vi "氨氮测量数据储存.vi"   [LabVIEW 2016, in "斯坦道氨氮.lvlib"]
types:
  T1 = cluster{"时间标识":timestamp, "监测值":sgl, "单位":u16, "数据标识":string, "因子编码":u32, "标样参考值":sgl, "F0":sgl, "F1":sgl, "F2":sgl, "F3":sgl, "F4":sgl, "F5":sgl, "F6":sgl, "F7":sgl, "X":sgl, "温度":sgl, "湿度":sgl, "量程标识":string}
  T2 = enum16{"维护数据", "水样测试", "标样核查", "零点核查", "跨度核查", "空白测试", "平行样测试", "加标回收", "空白校准", "标样校准", "初始化（清洗）"}
  T3 = cluster{"运行模式":enum16{"维护模式", "常规模式", "应急模式", "质控模式"}, "质控频次":enum16{"关闭", "每天", "星期一", "星期二", "星期三", "星期四", "星期五", "星期六", "星期日"}, "空白核查时间":u16, "跨度核查时间":u16, "24H周期设置":bool[]}
  T4 = cluster{"系统时间":timestamp, "工作状态":enum16{"空闲", "水样测试", "标样核查", "零点核查", "跨度核查", "空白测试", "平行样测试", "加标回收", "空白校准", "标样校准", "初始化（清洗）"}, "测量模式":enum16{"待机", "连续模式", "周期模式", "定点模式", "受控模式", "手动模式"}, "告警代码":enum16{"无告警", "缺试剂告警", "缺水样告警", "缺蒸馏水告警", "缺标液告警", "仪表漏液告警", "标定异常告警", "超量程告警", "加热异常", "低试剂预警", "超上限告警", "超下限告警", "仪表内部其他异常", "滴定异常告警", "电极异常告警", "量程切换告警", "参数设置告警", "PH电极电位异常", "电导率电极异常", "浊度光度异常", "溶解氧电极异常", "溶解氧光强异常", "温度异常告警", "PH异常告警", "溶解氧异常告警", "电导率异常告警", "浊度异常告警", "叶绿素异常告警", "藻密度异常告警", "蓝绿藻异常告警", "ORP异常告警", "氨氮异常告警", "清洁刷异常告警", "SD卡异常告警", "蓝牙异常告警", "Wifi异常告警", "流程异常告警"}, "故障代码":enum16{"无故障", "电机故障", "温度故障", "通讯故障", "滴定故障"}, "日志代码":u16, "软件版本":u16, "F0":sgl, "F1":sgl, "F2":sgl, "F3":sgl, "T":sgl, "H":sgl, "id":u16, "flowid":u16, "量程":u16, "总磷控温温度1":sgl, "营养盐控温温度2":sgl, "ADC":sgl}
  T5 = enum16{"空闲", "水样测试", "标样核查", "零点核查", "跨度核查", "空白测试", "平行样测试", "加标回收", "空白校准", "标样校准", "初始化（清洗）"}
  T6 = cluster{"因子编码":u32, "单位":u16, "标样参考值":sgl, "水样数据时间":timestamp, "水样实测值":sgl, "水样数据标识":string, "标样数据时间":timestamp, "标样实测值":sgl, "标样数据标识":string, "空白数据时间":timestamp, "空白实测值":sgl, "空白数据标识":string, "零点核查数据时间":timestamp, "零点核查实测值":sgl, "零点核查数据标识":string, "跨度核查数据时间":timestamp, "跨度核查实测值":sgl, "跨度核查数据标识":string, "加标回收数据时间":timestamp, "加标回收实测值":sgl, "加标回收数据标识":string, "平行样数据时间":timestamp, "平行样实测值":sgl, "平行样数据标识":string, "F0":sgl, "F1":sgl, "F2":sgl, "F3":sgl, "F4":sgl, "F5":sgl, "F6":sgl, "F7":sgl, "温度":sgl, "湿度":sgl, "X值":sgl}
  T7 = cluster{"氨氮跨度值":dbl, "氨氮零点标准液浓度":dbl, "氨氮跨度标准液浓度":dbl, "氨氮标准液标准浓度":dbl}
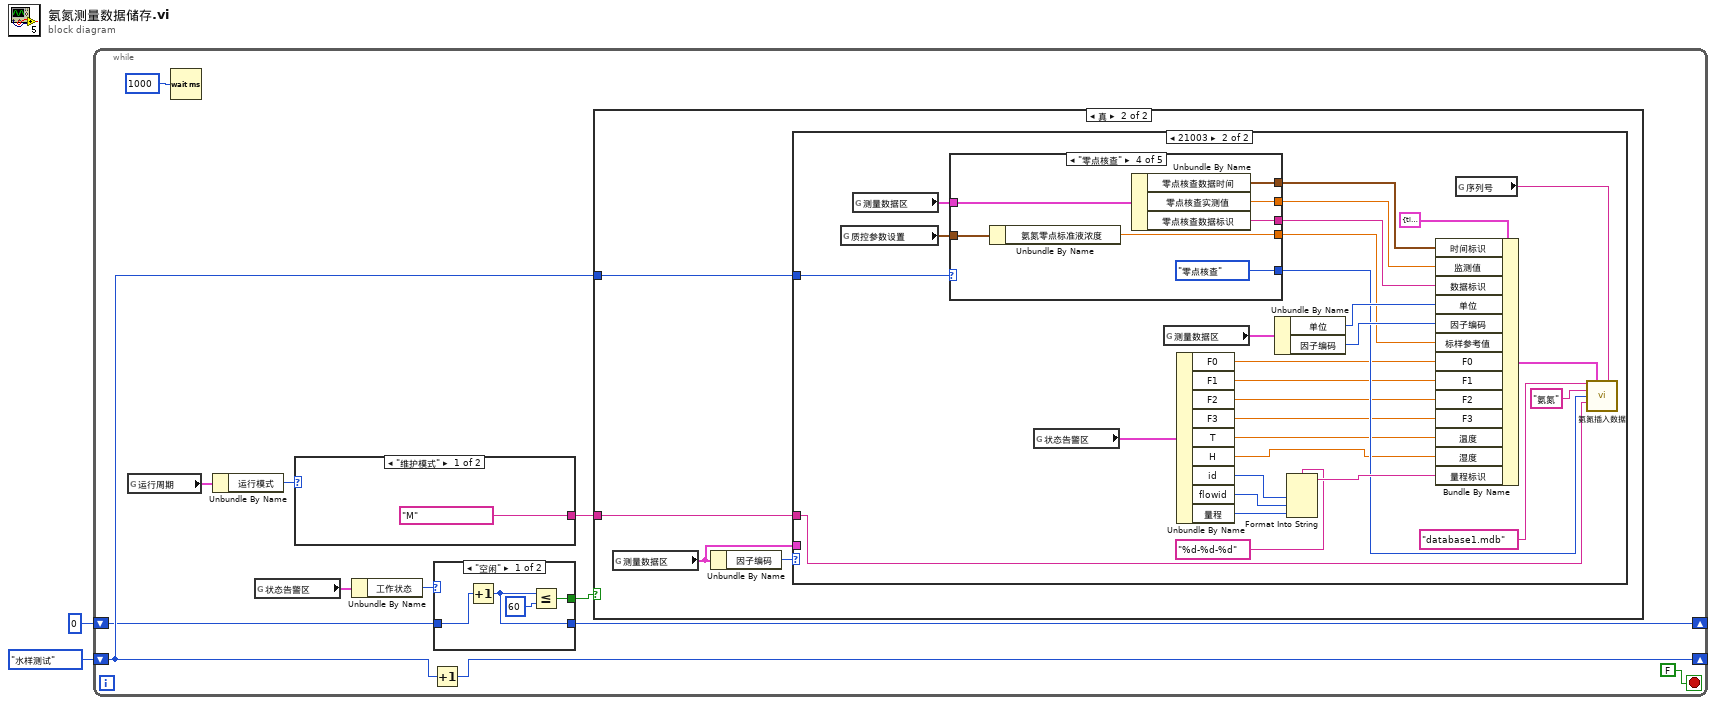
[diagram p0: block diagram]
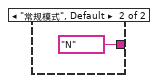
[diagram p3: hidden frame]
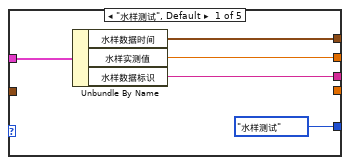
[diagram p6: hidden frame]
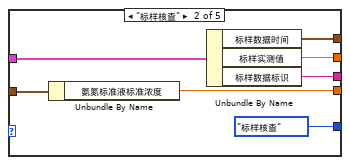
[diagram p7: hidden frame]
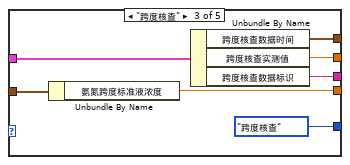
[diagram p8: hidden frame]
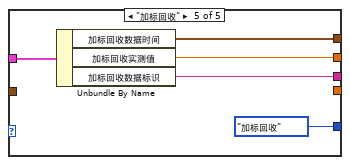
[diagram p9: hidden frame]
diagram:
  n1 = while {
    shift-right: [w11] -> _
    shift-left: enum16{"水样测试", "标样核查", "跨度核查", "零点核查", "加标回收"}."水样测试" ("测量模式") -> [w10]
    shift-right: [w4] -> _
    shift-left: u32 0 ("等待时间（毫秒）") -> [w5]
    stop <- FALSE stop-if-true
    n2 = global read "氨氮断电保存全局变量.vi" "运行周期"() -> (w9:T3)
    n3 = Wait (ms)(milliseconds to wait=u32 1000 ("等待时间（毫秒）")) -> ()  [unwired: 1 out]
    n4 = Unbundle By Name(w9) -> ("运行模式"=w8:enum16{"维护模式", "常规模式", "应急模式", "质控模式"})
    n5 = global read "VAR氨氮全局变量.vi" "状态告警区"() -> (w7:T4)
    n6 = case shown="\"维护模式\"" w8 {
      tunnel: ["M" ("数据标记表") "N" ("数据标记表")] -> w12
      frame "维护模式" {
      }
      frame "常规模式", Default {
      }
    }
    n7 = Unbundle By Name(w7) -> ("工作状态"=w6:T5)
    n8 = Increment(x=w10) -> (x+1=w11:enum16{"水样测试", "标样核查", "跨度核查", "零点核查", "加标回收"})
    n9 = case shown="\"空闲\"" w6 {
      tunnel: w5 -> [w18 _]
      tunnel: [w17 _] -> w4
      tunnel: [w15 _] -> w3
      frame "空闲" {
        n10 = Increment(x=w18) -> (x+1=w17:u32)
        n11 = Less Or Equal?(x=w17, y=u32 60) -> (x <= y?=w15:bool)
      }
      frame "水样测试", Default {
      }
    }
    n12 = case shown="真" w3 {
      tunnel: w12 -> [_ w22]
      tunnel: w10 -> [_ w21]
      frame False {
      }
      frame True {
        n13 = global read "VAR氨氮全局变量.vi" "测量数据区"() -> (w24:T6)
        n14 = Unbundle By Name(w24) -> ("因子编码"=w23:u32)
        n15 = case shown="21003" w23 {
          tunnel: w24 -> [_ _]
          tunnel: w22 -> [_ w35]
          tunnel: w21 -> [_ w34]
          frame Default {
          }
          frame 21003 {
            n16 = global read "氨氮断电保存全局变量.vi" "质控参数设置"() -> (w32:T7)
            n17 = global read "VAR氨氮全局变量.vi" "测量数据区"() -> (w52:T6)
            n18 = case shown="\"零点核查\"" w34 {
              tunnel: w52 -> [w58 w65 w72 w79 w84]
              tunnel: [w57 w64 w71 w78 w83] -> w39
              tunnel: [w56 w63 w70 w77 w82] -> w40
              tunnel: [w55 w62 w69 w76 w81] -> w41
              tunnel: [T2."水样测试" ("测量模式") T2."标样核查" ("测量模式") T2."跨度核查" ("测量模式") T2."零点核查" ("测量模式") T2."加标回收" ("测量模式")] -> w38
              tunnel: w32 -> [_ w60 w67 w74 _]
              tunnel: [_ w59 w66 w73 _] -> w31
              frame "水样测试", Default {
                n19 = Unbundle By Name(w58) -> ("水样数据时间"=w57:timestamp, "水样实测值"=w56:sgl, "水样数据标识"=w55:string)
              }
              frame "标样核查" {
                n20 = Unbundle By Name(w60) -> ("氨氮标准液标准浓度"=w59:dbl)
                n21 = Unbundle By Name(w65) -> ("标样数据时间"=w64:timestamp, "标样实测值"=w63:sgl, "标样数据标识"=w62:string)
              }
              frame "跨度核查" {
                n22 = Unbundle By Name(w67) -> ("氨氮跨度标准液浓度"=w66:dbl)
                n23 = Unbundle By Name(w72) -> ("跨度核查数据时间"=w71:timestamp, "跨度核查实测值"=w70:sgl, "跨度核查数据标识"=w69:string)
              }
              frame "零点核查" {
                n24 = Unbundle By Name(w74) -> ("氨氮零点标准液浓度"=w73:dbl)
                n25 = Unbundle By Name(w79) -> ("零点核查数据时间"=w78:timestamp, "零点核查实测值"=w77:sgl, "零点核查数据标识"=w76:string)
              }
              frame "加标回收" {
                n26 = Unbundle By Name(w84) -> ("加标回收数据时间"=w83:timestamp, "加标回收实测值"=w82:sgl, "加标回收数据标识"=w81:string)
              }
            }
            n27 = global read "VAR氨氮全局变量.vi" "状态告警区"() -> (w33:T4)
            n28 = global read "VAR氨氮全局变量.vi" "测量数据区"() -> (w46:T6)
            n29 = Unbundle By Name(w33) -> ("F0"=w30:sgl, "F1"=w29:sgl, "F2"=w28:sgl, "F3"=w27:sgl, "T"=w26:sgl, "H"=w25:sgl, "id"=w53:u16, "flowid"=w48:u16, "量程"=w47:u16)
            n30 = Unbundle By Name(w46) -> ("单位"=w51:u16, "因子编码"=w50:u32)
            n31 = Format Into String(format string="%d-%d-%d" ("格式字符串"), w53, w48, w47) -> (resulting string=w49:string)  [unwired: 2 in, 1 out]
            n32 = Bundle By Name(cluster=T1 {"时间标识"=timestamp(0 s since 1904-01-01), "监测值"=0.0, "单位"=0, "数据标识"="", "因子编码"=0, "标样参考值"=0.0, "F0"=0.0, "F1"=0.0, "F2"=0.0, "F3"=0.0, "F4"=0.0, "F5"=0.0, "F6"=0.0, "F7"=0.0, "X"=0.0, "温度"=0.0, "湿度"=0.0, "量程标识"=""} ("data"), "时间标识"=w39, "监测值"=w40, "数据标识"=w41, "单位"=w51, "因子编码"=w50, "标样参考值"=w31, "F0"=w30, "F1"=w29, "F2"=w28, "F3"=w27, "温度"=w26, "湿度"=w25, "量程标识"=w49) -> (w43:T1)
            n33 = global read "VAR氨氮全局变量.vi" "序列号"() -> (w42:string)
            n34 = call "氨氮插入数据.vi"("database"="database1.mdb", "data"=w43, "SN"=w42, "table"="氨氮", "测量模式"=w38, "数据标记表"=w35) -> ()  [unwired: 9 in, 1 out]
          }
        }
      }
    }
  }
